vi "PM100D Simple Example - 複製.vi"() -> ()   [LabVIEW 2014]
doc: "This VI shows how to communicate with a PM100D optical power/energy meter with SCPI commands.\n- Initializing the instrument\n- Getting system info\n- Setting parameters\n- Measurement configuration\n- Measuring queue\n- Fetching and displaying a measurement value\n- Closing the application"
panel:
  out "Readout value":dbl format="%^#_9e"
  out "IDN String":string
  out "Sensor SN":string
  out "Sensor Name":string
  out "Sensor Flags":bool[](array[boolean])
  out "New":bool
  in  "Timeout [ms]":i32=1000
  in  "stop":bool
  in  "Readout Config":string(combo)="POW"
  out "Readout string":string
  out "Error log":string
  in  "Averaging Rate":i32=300
  # "1 Power Sensor"
  # "2 Energy Sensor"
  # "4"
  # "8"
  # "16 Response settable"
  # "32 Wavelength settable"
  # "64 Tau (time constant) settable"
  # "128"
  # "256 With temperature sensor"
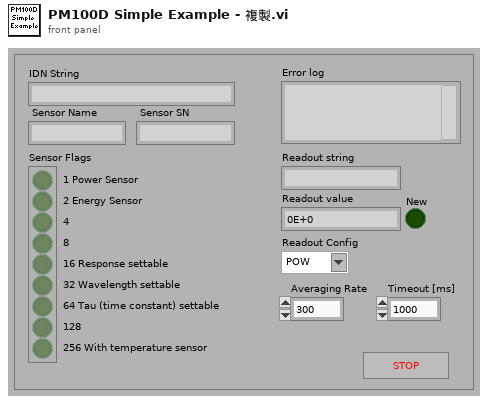
[diagram p1: front panel]
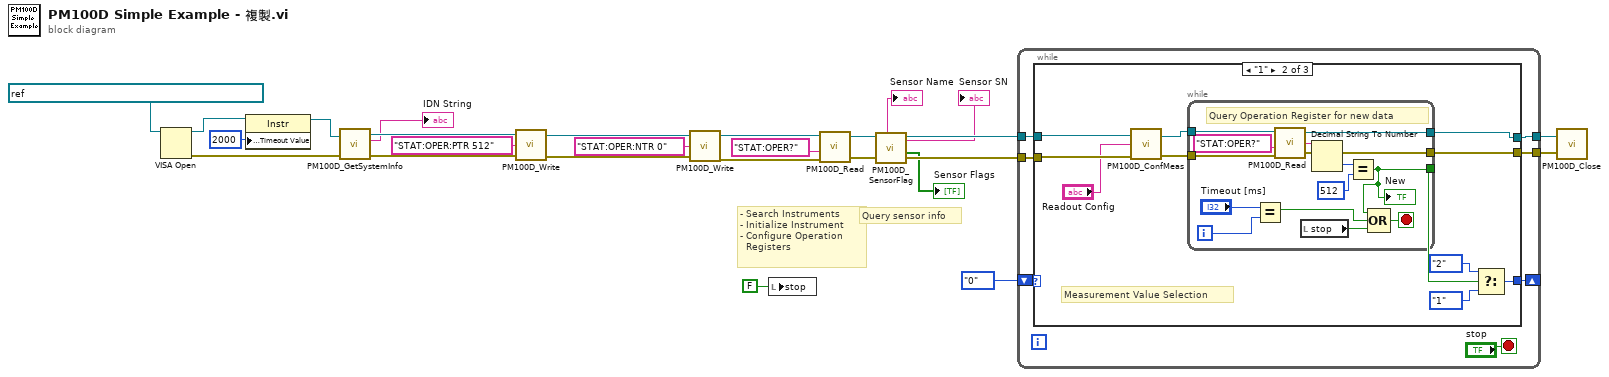
[diagram p0: block diagram]
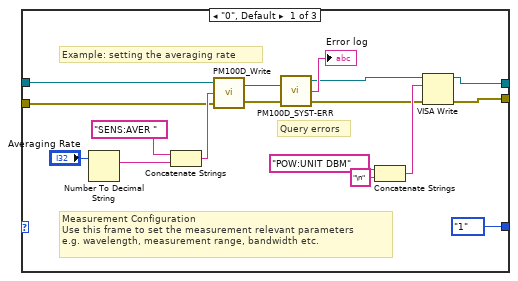
[diagram p2: hidden frame]
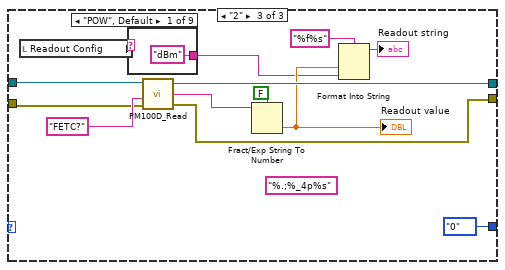
[diagram p3: hidden frame]
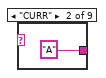
[diagram p4: hidden frame]
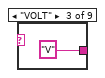
[diagram p5: hidden frame]
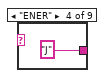
[diagram p6: hidden frame]
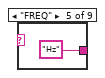
[diagram p7: hidden frame]
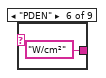
[diagram p8: hidden frame]
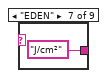
[diagram p9: hidden frame]
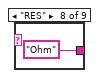
[diagram p10: hidden frame]
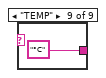
[diagram p11: hidden frame]
diagram:
  # "- Search Instruments\n- Initialize Instrument\n- Configure Operation\n  Registers"
  # "Query sensor info"
  n1 = VISA Open(VISA resource name=refnum<visa-resource-name> "USB0::0x1313::0x8078::P0027168::INSTR") -> (VISA resource name=w15:refnum<visa-resource-name>, error out=w17:errorcluster)  [unwired: 1 in, 3 out]
  n2 = property class="Instr"(reference=w15, "General Settings:Timeout Value"=u32 2000) -> (reference out=w14:refnum<visa-resource-name>)  [unwired: 1 in, 1 out]
  n3 = call "PM100D_GetSystemInfo.vi"("VISA in"=w14, "error in"=w17) -> ("VISA out"=w12:refnum<visa-resource-name>, "Instrument"=→"IDN String":string, "error out"=w10:errorcluster)  [unwired: 1 out]
  n4 = call "PM100D_Write.vi"("error in (no error)"=w10, "Command"="STAT:OPER:PTR 512", "VISA in"=w12) -> ("error out"=w9:errorcluster, "VISA out"=w11:refnum<visa-resource-name>)
  n5 = call "PM100D_Write.vi"("error in (no error)"=w9, "Command"="STAT:OPER:NTR 0", "VISA in"=w11) -> ("error out"=w5:errorcluster, "VISA out"=w7:refnum<visa-resource-name>)
  n6 = local write "stop"(FALSE ("stop")) -> ()
  n7 = call "PM100D_Read.vi"("error in (no error)"=w5, "Command"="STAT:OPER?", "VISA in"=w7) -> ("error out"=w1:errorcluster, "VISA out"=w2:refnum<visa-resource-name>)  [unwired: 1 in, 1 out]
  n8 = call "PM100D_SensorFlag.vi"("error in (no error)"=w1, "VISA in"=w2) -> ("error out"=w25:errorcluster, "flags"=→"Sensor Flags":bool[], "VISA out"=w26:refnum<visa-resource-name>, "sn"=→"Sensor SN":string, "name"=→"Sensor Name":string)  [unwired: 2 in, 3 out]
  n9 = while {
    tunnel: w26 -> [w33]
    tunnel: w25 -> [w32]
    shift-right: [w29] -> _
    shift-left: enum16{"0", "1", "2"}."0" -> [w30]
    tunnel: [w28] -> w20
    tunnel: [w27] -> w19
    stop <- "stop" stop-if-true
    n10 = case shown="\"1\"" w30 {
      tunnel: w33 -> [w47 w61 w86]
      tunnel: w32 -> [w42 w60 w85]
      tunnel: [enum16{"0", "1", "2"}."1" w55 enum16{"0", "1", "2"}."0"] -> w29
      tunnel: [w37 w57 w84] -> w28
      tunnel: [w36 w56 w76] -> w27
      frame "0", Default {
        # "Query errors"
        # "Example: setting the averaging rate"
        # "Measurement Configuration\nUse this frame to set the measurement relevant parameters\ne.g. wavelength, measurement range, bandwidth etc."
        n11 = Number To Decimal String(number="Averaging Rate") -> (decimal integer string=w49:string)  [unwired: 1 in]
        n12 = Concatenate Strings("SENS:AVER " ("string"), w49) -> (w46:string)
        n13 = call "PM100D_Write.vi"("error in (no error)"=w42, "Command"=w46, "VISA in"=w47) -> ("error out"=w43:errorcluster, "VISA out"=w45:refnum<visa-resource-name>)
        n14 = call "PM100D_SYST-ERR.vi"("error out 2"=w43, "VISA In"=w45) -> ("error out"=w34:errorcluster, "Error"=→"Error log":string, "VISA Out"=w35:refnum<visa-resource-name>)  [unwired: 1 in]
        n15 = Concatenate Strings("POW:UNIT DBM" ("string"), "\n" ("String")) -> (w38:string)
        n16 = VISA Write(VISA resource name=w35, write buffer=w38, error in (no error)=w34) -> (VISA resource name out=w37:refnum<visa-resource-name>, error out=w36:errorcluster)  [unwired: 1 out]
      }
      frame "1" {
        # "Measurement Value Selection"
        n17 = call "PM100D_ConfMeas.vi"("error in"=w60, "Conf:"="Readout Config", "VISA In"=w61) -> ("error out"=w58:errorcluster, "dup VISA session"=w59:refnum<visa-resource-name>)
        n18 = while {
          tunnel: w59 -> [w71]
          tunnel: w58 -> [w70]
          tunnel: [w69] -> w57
          tunnel: [w68] -> w56
          tunnel: [w62] -> w52
          i -> [w64]
          stop <- w66 stop-if-true
          # "Query Operation Register for new data"
          n19 = Equal?(x="Timeout [ms]", y=w64) -> (x = y?=w63:bool)
          n20 = call "PM100D_Read.vi"("error in (no error)"=w70, "Command"="STAT:OPER?", "VISA in"=w71) -> ("error out"=w68:errorcluster, "ReadValue"=w74:string, "VISA out"=w69:refnum<visa-resource-name>)  [unwired: 1 in]
          n21 = local read "stop"() -> (w67:bool)
          n22 = Decimal String To Number(string=w74) -> (number=w73:i32)  [unwired: 2 in, 1 out]
          n23 = Equal?(x=w73, y=512) -> (x = y?=w62:bool)
          "New" <- w62
          n24 = Compound Arithmetic op=OR(w62, w63, w67) -> (w66:bool)
        }
        n25 = Select(t=enum16{"0", "1", "2"}."2", s=w52, f=enum16{"0", "1", "2"}."1") -> (s? t:f=w55:enum16{"0", "1", "2"})
      }
      frame "2" {
        (unwired) "%.;%_4p%s" ("format string")
        n26 = local read "Readout Config"() -> (w83:string)
        n27 = case shown="\"POW\", Default" w83 {
          tunnel: ["dBm" "A" "V" "J" "Hz" "W/cm²" "J/cm²" "Ohm" "°C"] -> w78
          frame "POW", Default {
          }
          frame "CURR" {
          }
          frame "VOLT" {
          }
          frame "ENER" {
          }
          frame "FREQ" {
          }
          frame "PDEN" {
          }
          frame "EDEN" {
          }
          frame "RES" {
          }
          frame "TEMP" {
          }
        }
        n28 = call "PM100D_Read.vi"("error in (no error)"=w85, "Command"="FETC?", "VISA in"=w86) -> ("error out"=w76:errorcluster, "ReadValue"=w82:string, "VISA out"=w84:refnum<visa-resource-name>)  [unwired: 1 in]
        n29 = Fract/Exp String To Number(use system decimal point (T)=FALSE, string=w82) -> (number=w79:dbl)  [unwired: 2 in, 1 out]
        "Readout value" <- w79
        n30 = Format Into String(format string="%f%s", w79, w78) -> (resulting string=→"Readout string":string)  [unwired: 2 in, 1 out]
      }
    }
  }
  n31 = call "PM100D_Close.vi"("error in (no error)"=w19, "VISA resource name"=w20) -> ()  [unwired: 1 in, 1 out]
